vi "ep_Public Inf to Task.vi"(7 "include config info? (F)":bool, 8 "error in":errorcluster, 9 "public event information":T1[](array[typedef]) {"min sample number" max=9999999999; "max sample number" max=9999999999}, 10 "public record information":T2={"source"="", "record type"=enum."Unknown", "phase ID"="", "event description"="", "device ID"="", "distance of fault"=-1.0, "distance unit"=enum."Miles", "max current"=-inf, "min current"=inf, "max voltage"=-inf, "min voltage"=inf}, 11 "task in":T3={"file refnums"=[], "Data Object"=refnum, "config info"={"station_name"="", "rec_dev_id"="", "rev_year"=1999.0, "TT"=0, "##A"=0, "##D"=0, "analog channel info"=[], "status channel info"=[], "lf"=50.0, "nrates"=0, "samp info"=[], "initial timestamp"=timestamp(0 s since 1904-01-01), "trigger timestamp"=timestamp(0 s since 1904-01-01), "ft"=enum."Binary", "timemult"=1.0}, "public inf content"={"Source"="", "Record Type"=enum."Unknown", "Phase ID"="", "Event Description"="", "Device ID"="", "Distance of Fault"=-1.0, "Distance Unit"=enum."Miles", "Max_Current"=-inf, "Min_Current"=inf, "Max_Voltage"=-inf, "Min_Voltage"=inf, "EventNoteCount"=0, "Event Information"=[]}, "private inf content"=[], "internal buffers"={"start index"=1, "config to public inf"=enum."disabled", "static config info"="", "static file_des record inf"="", "static file_des channel inf"="", "public inf"="", "private inf"=""}} {"public inf content"."Event Information"."min sample number" max=9999999999; "public inf content"."Event Information"."max sample number" max=9999999999; "config info"."nrates" max=999; "config info"."status channel info"."Dn" min=1 max=999999; "config info"."analog channel info"."An" min=1 max=999999; "config info"."trigger timestamp" format="%<%H:%M:%S%6u\n%d/%m/%Y>T"; "config info"."initial timestamp" format="%<%H:%M:%S%6u\n%d/%m/%Y>T"; "config info"."##D" max=999999; "config info"."##A" max=999999; "config info"."TT" min=1 max=999999; "config info"."rev_year" min=1999.0 max=1999.0}) -> (0 "error out":errorcluster, 3 "task out":T3={"file refnums"=[], "Data Object"=refnum, "config info"={"station_name"="", "rec_dev_id"="", "rev_year"=1999.0, "TT"=0, "##A"=0, "##D"=0, "analog channel info"=[], "status channel info"=[], "lf"=50.0, "nrates"=0, "samp info"=[], "initial timestamp"=timestamp(0 s since 1904-01-01), "trigger timestamp"=timestamp(0 s since 1904-01-01), "ft"=enum."Binary", "timemult"=1.0}, "public inf content"={"Source"="", "Record Type"=enum."Unknown", "Phase ID"="", "Event Description"="", "Device ID"="", "Distance of Fault"=-1.0, "Distance Unit"=enum."Miles", "Max_Current"=-inf, "Min_Current"=inf, "Max_Voltage"=-inf, "Min_Voltage"=inf, "EventNoteCount"=0, "Event Information"=[]}, "private inf content"=[], "internal buffers"={"start index"=1, "config to public inf"=enum."disabled", "static config info"="", "static file_des record inf"="", "static file_des channel inf"="", "public inf"="", "private inf"=""}} {"public inf content"."Event Information"."min sample number" max=9999999999; "public inf content"."Event Information"."max sample number" max=9999999999; "config info"."nrates" max=999; "config info"."status channel info"."Dn" min=1 max=999999; "config info"."analog channel info"."An" min=1 max=999999; "config info"."trigger timestamp" format="%<%H:%M:%S%6u\n%d/%m/%Y>T"; "config info"."initial timestamp" format="%<%H:%M:%S%6u\n%d/%m/%Y>T"; "config info"."##D" max=999999; "config info"."##A" max=999999; "config info"."TT" min=1 max=999999; "config info"."rev_year" min=1999.0 max=1999.0})   [LabVIEW 2011, in "NI_EP_COMTRADE.lvlib"]
uses:
  <vilib>/addons/Electrical Power/File IO/NI_EP_COMTRADE.lvlib
  <vilib>/addons/Electrical Power/File IO/COMTRADE/typedefs/ep_Task.ctl
  <vilib>/addons/Electrical Power/File IO/COMTRADE/typedefs/ep_Config Info.ctl
  <vilib>/addons/Electrical Power/File IO/COMTRADE/typedefs/ep_Analog Channel Info.ctl
  <vilib>/addons/Electrical Power/File IO/COMTRADE/typedefs/ep_Status Channel Info.ctl
  <vilib>/addons/Electrical Power/File IO/COMTRADE/typedefs/ep_File Format.ctl
  <vilib>/addons/Electrical Power/File IO/COMTRADE/typedefs/ep_Public Inf Content.ctl
  <vilib>/addons/Electrical Power/File IO/COMTRADE/typedefs/ep_Public Event Inf.ctl
  <vilib>/addons/Electrical Power/File IO/COMTRADE/typedefs/ep_Private Inf Content.ctl
  <vilib>/addons/Electrical Power/File IO/COMTRADE/typedefs/ep_Public Record Inf.ctl
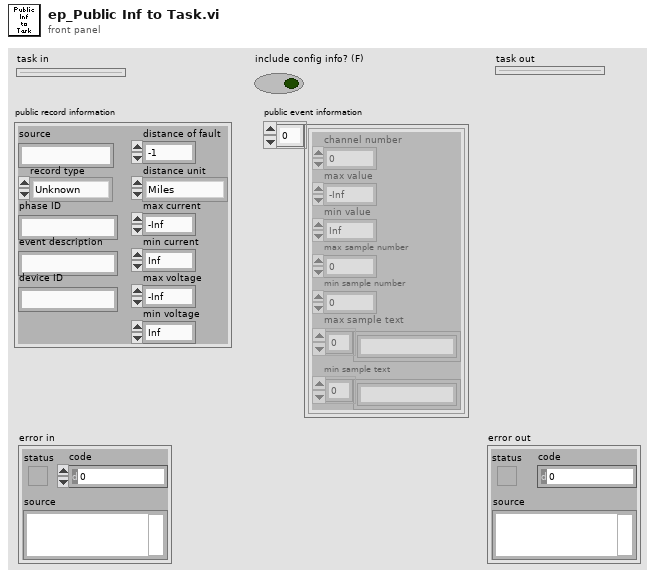
[diagram p1: front panel]
types:
  T1 = typedef "NI_EP_COMTRADE.lvlib/ep_Public Event Inf.ctl" = cluster{"channel number":u32, "max value":dbl, "min value":dbl, "max sample number":u64, "min sample number":u64, "max sample text":string[], "min sample text":string[]}
  T2 = typedef "NI_EP_COMTRADE.lvlib/ep_Public Record Inf.ctl" = cluster{"source":string, "record type":enum16{"Fault", "Unknown", "Misoperation", "Close", "Trip", "Reclose", "Power swing", "Simulation"}, "phase ID":string, "event description":string, "device ID":string, "distance of fault":dbl, "distance unit":enum16{"Miles", "Kilometers", "Percent of line", "Percent of setting", "Ohms"}, "max current":dbl, "min current":dbl, "max voltage":dbl, "min voltage":dbl}
  T3 = typedef "NI_EP_COMTRADE.lvlib/ep_Task.ctl" = cluster{"file refnums":refnum<file>[], "Data Object":refnum<k20>, "config info":T4, "public inf content":T8, "private inf content":T9, "internal buffers":cluster{"start index":u32, "config to public inf":enum16{"disabled", "enabled", "buffered"}, "static config info":string, "static file_des record inf":string, "static file_des channel inf":string, "public inf":string, "private inf":string}}
  T4 = typedef "NI_EP_COMTRADE.lvlib/ep_Config Info.ctl" = cluster{"station_name":string, "rec_dev_id":string, "rev_year":dbl, "TT":u32, "##A":u32, "##D":u32, "analog channel info":T5[], "status channel info":T6[], "lf":sgl, "nrates":u16, "samp info":cluster{"samp":sgl, "endsamp":u32}[], "initial timestamp":timestamp, "trigger timestamp":timestamp, "ft":T7, "timemult":sgl}
  T5 = typedef "NI_EP_COMTRADE.lvlib/ep_Analog Channel Info.ctl" = cluster{"An":u32, "ch_id":string, "ph":string, "ccbm":string, "uu":string, "a":sgl, "b":sgl, "skew":sgl, "min":i32, "max":i32, "primary":sgl, "secondary":sgl, "PS":enum16{"P", "S"}}
  T6 = typedef "NI_EP_COMTRADE.lvlib/ep_Status Channel Info.ctl" = cluster{"Dn":u32, "ch_id":string, "ph":string, "ccbm":string, "Y":bool}
  T7 = typedef "NI_EP_COMTRADE.lvlib/ep_File Format.ctl" = enum16{"ASCII", "Binary"}
  T8 = typedef "NI_EP_COMTRADE.lvlib/ep_Public Inf Content.ctl" = cluster{"Source":string, "Record Type":enum16{"Fault", "Unknown", "Misoperation", "Close", "Trip", "Reclose", "Power swing", "Simulation"}, "Phase ID":string, "Event Description":string, "Device ID":string, "Distance of Fault":dbl, "Distance Unit":enum16{"Miles", "Kilometers", "Percent of line", "Percent of setting", "Ohms"}, "Max_Current":dbl, "Min_Current":dbl, "Max_Voltage":dbl, "Min_Voltage":dbl, "EventNoteCount":u32, "Event Information":T1[]}
  T9 = typedef "NI_EP_COMTRADE.lvlib/ep_Private Inf Content.ctl" = cluster{"Section Header":string, "Entry Names":string[], "Entry Values":string[]}[]
  T10 = enum16{"Fault", "Unknown", "Misoperation", "Close", "Trip", "Reclose", "Power swing", "Simulation"}
  T11 = enum16{"Miles", "Kilometers", "Percent of line", "Percent of setting", "Ohms"}
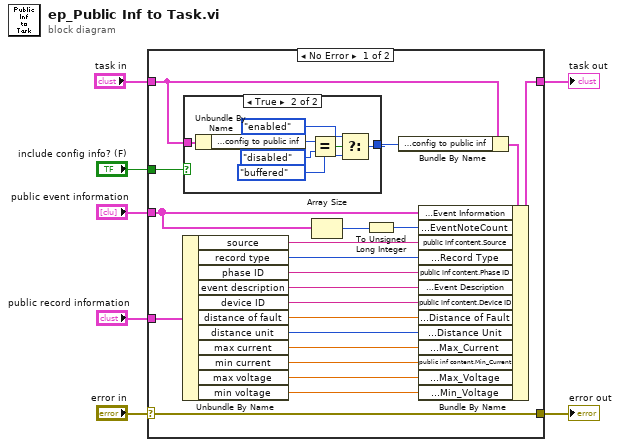
[diagram p0: block diagram]
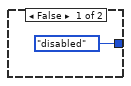
[diagram p2: hidden frame]
diagram:
  n1 = case shown="No Error" "error in" {
    selector: "error in" -> [w10 w37]
    tunnel: "task in" -> [w14 w38]
    tunnel: [w9 w38] -> w5
    tunnel: [w10 w37] -> w4
    tunnel: "public record information" -> [w28 _]
    tunnel: "include config info? (F)" -> [w16 _]
    tunnel: "public event information" -> [w8 _]
    frame No Error {
      n2 = Unbundle By Name(w28) -> ("source"=w27:string, "record type"=w26:T10, "phase ID"=w25:string, "event description"=w24:string, "device ID"=w23:string, "distance of fault"=w22:dbl, "distance unit"=w21:T11, "max current"=w20:dbl, "min current"=w19:dbl, "max voltage"=w18:dbl, "min voltage"=w17:dbl)
      n3 = case shown="True" w16 {
        tunnel: [enum16{"disabled", "enabled", "buffered"}."disabled" ("internal buffers.config to public inf") w31] -> w15
        tunnel: w14 -> [_ w30]
        frame False {
        }
        frame True {
          n4 = Unbundle By Name(w30) -> ("internal buffers.config to public inf"=w36:enum16{"disabled", "enabled", "buffered"})
          n5 = Equal?(x=w36, y=enum16{"disabled", "enabled", "buffered"}."disabled" ("internal buffers.config to public inf")) -> (x = y?=w34:bool)
          n6 = Select(t=enum16{"disabled", "enabled", "buffered"}."enabled" ("internal buffers.config to public inf"), s=w34, f=enum16{"disabled", "enabled", "buffered"}."buffered" ("internal buffers.config to public inf")) -> (s? t:f=w31:enum16{"disabled", "enabled", "buffered"})
        }
      }
      n7 = Array Size(array=w8) -> (size(s)=w12:i32)
      n8 = To Unsigned Long Integer(number=w12) -> (unsigned 32bit integer=w11:u32)
      n9 = Bundle By Name(cluster=w14, "internal buffers.config to public inf"=w15) -> (w13:T3)
      n10 = Bundle By Name(cluster=w13, "public inf content.Event Information"=w8, "public inf content.EventNoteCount"=w11, "public inf content.Source"=w27, "public inf content.Record Type"=w26, "public inf content.Phase ID"=w25, "public inf content.Event Description"=w24, "public inf content.Device ID"=w23, "public inf content.Distance of Fault"=w22, "public inf content.Distance Unit"=w21, "public inf content.Max_Current"=w20, "public inf content.Min_Current"=w19, "public inf content.Max_Voltage"=w18, "public inf content.Min_Voltage"=w17) -> (w9:T3)
    }
    frame Error {
    }
  }
  "task out" <- w5
  "error out" <- w4
